vi "Get Bytes.vi"(11 "MsgPackObject in":refnum<class "MsgPackObject.lvclass">) -> (2 "Array":u8[](array[numeric]), 3 "MsgPackObject out":refnum<class "MsgPackObject.lvclass">)   [LabVIEW 2020, in "wamplv.lvlib" / "MsgPackObject.lvclass"]
uses:
  MsgPackObject.lvclass
  MsgPackObject.lvclass/MsgPackObject.ctl
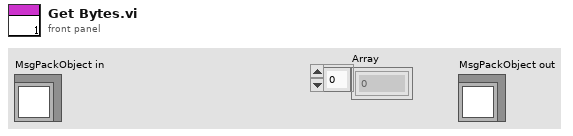
[diagram p1: front panel]
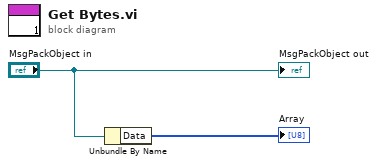
[diagram p0: block diagram]
diagram:
  n1 = Unbundle By Name("MsgPackObject in") -> ("Data"=→"Array":u8[])
  "MsgPackObject out" <- "MsgPackObject in"
